vi "Write XY unit scale factor.vi"(8 "error in (no error)":errorcluster, 10 "XY unit scale factor":dbl, 11 "XYCalFactor in":refnum<class "XYCalFactor.lvclass">) -> (0 "error out":errorcluster, 3 "XYCalFactor out":refnum<class "XYCalFactor.lvclass">)   [LabVIEW 2013, in "MaterialCharacterization.lvlib" / "XYCalFactor.lvclass"]
uses:
  XYCalFactor.lvclass
  XYCalFactor.lvclass/XYCalFactor.ctl
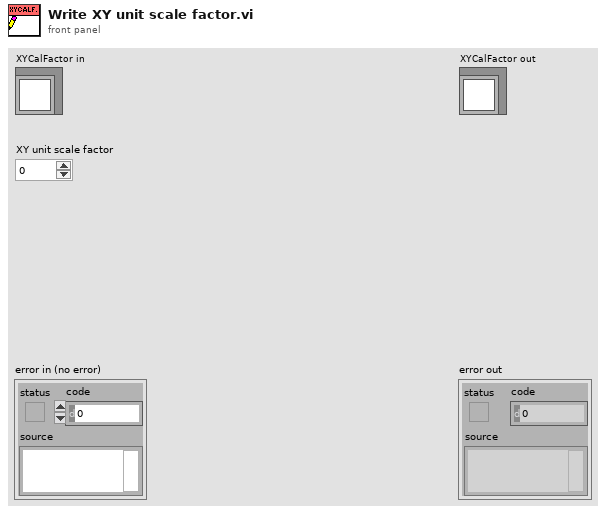
[diagram p1: front panel]
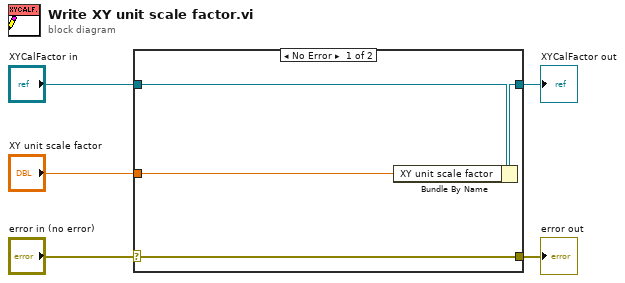
[diagram p0: block diagram]
diagram:
  n1 = case shown="No Error" "error in (no error)" {
    selector: "error in (no error)" -> [w9 w10]
    tunnel: [w9 w10] -> w4
    tunnel: [w7 w11] -> w2
    tunnel: "XYCalFactor in" -> [w8 w11]
    tunnel: "XY unit scale factor" -> [w6 _]
    frame No Error {
      n2 = Bundle By Name(cluster=w8, "XY unit scale factor"=w6) -> (w7:refnum<class "XYCalFactor.lvclass">)
    }
    frame Error {
    }
  }
  "error out" <- w4
  "XYCalFactor out" <- w2
